vi "PrepareGameData.vi"(8 "error in":errorcluster, 11 "GameDataIn":T1) -> (0 "error out":errorcluster, 3 "GameDataOut":T1)   [LabVIEW 2024]
uses:
  Controls/ArmySelector.ctl
  Controls/GameInfo.ctl
  Controls/E_Phases.ctl
  <vilib>/Utility/file.llb/Read Delimited Spreadsheet (string).vi
panel:
  in  "Opponent Army":T3
  in  "Player Army":T3
  out "String":string
  in  "Done":bool
  in  "LocationOfData":path
  in  "OpponentName":string
  in  "PlayerName":string
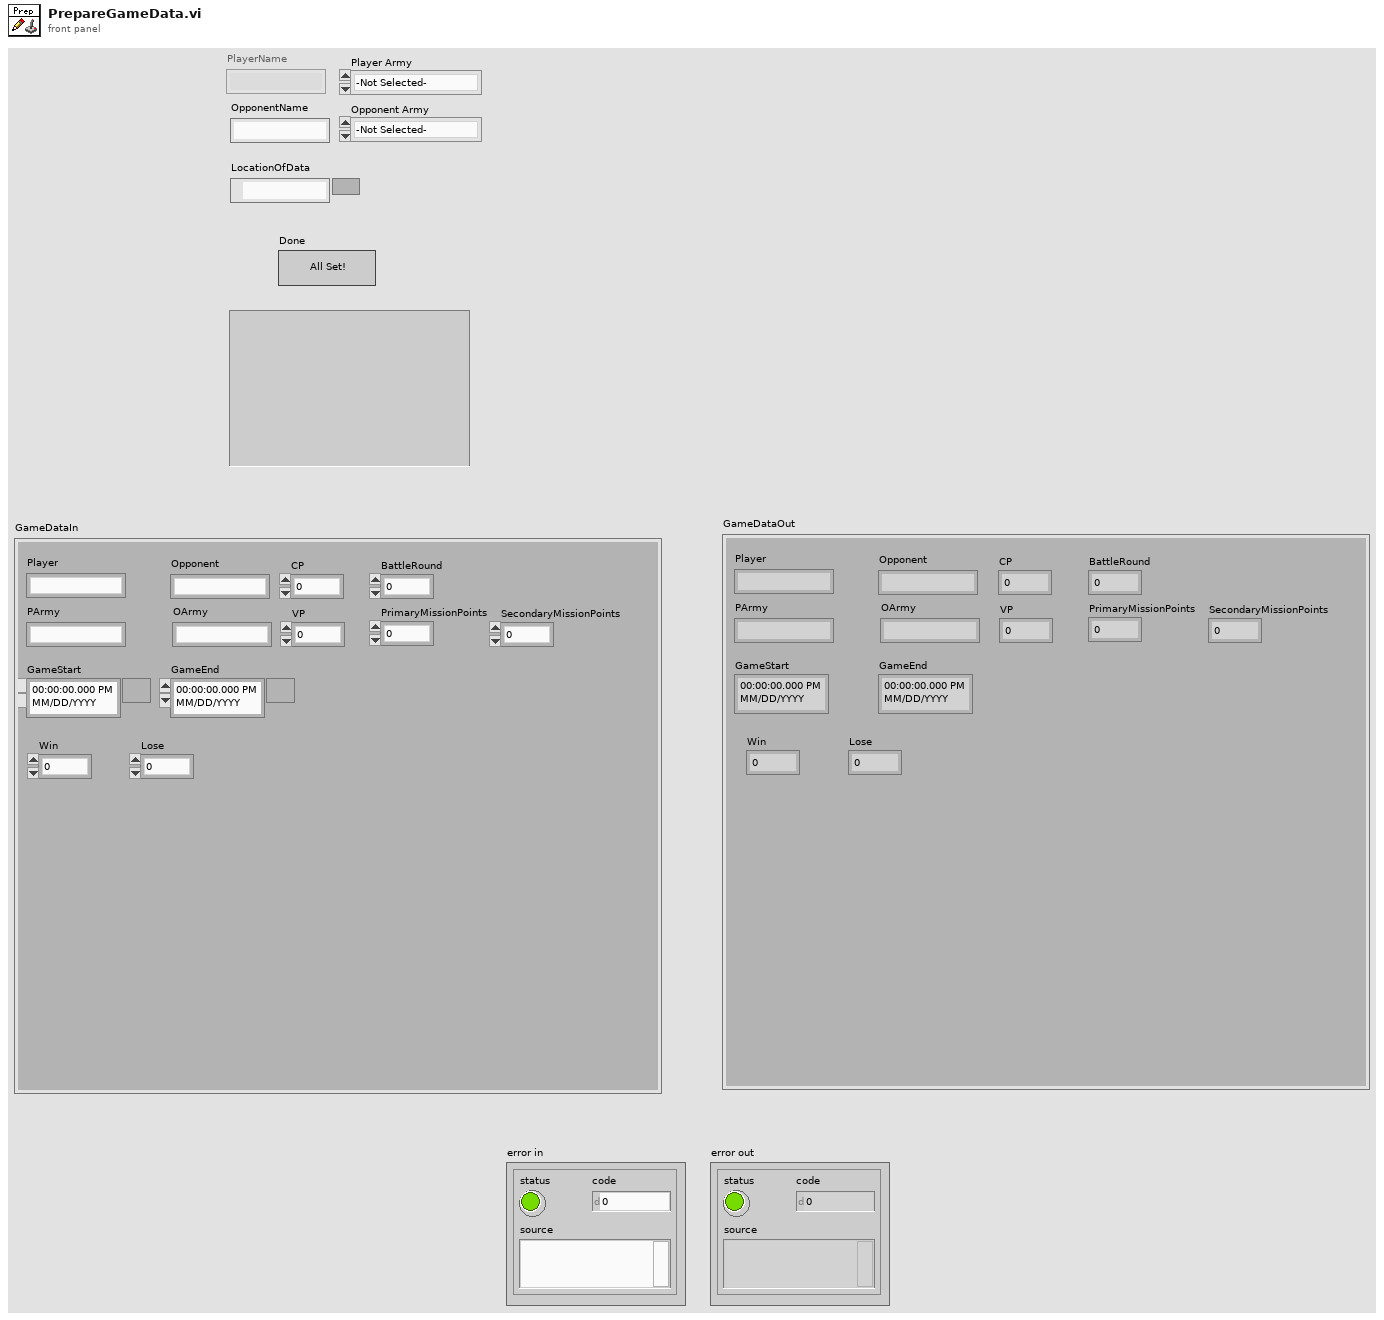
[diagram p1: front panel]
types:
  T1 = typedef "GameInfo.ctl" = cluster{"Player":string, "Opponent":string, "PArmy":string, "OArmy":string, "CP":dbl, "VP":dbl, "GameStart":timestamp, "GameEnd":timestamp, "BattleRound":dbl, "PrimaryMissionPoints":dbl, "SecondaryMissionPoints":dbl, "BattlePhase":T2, "Win":dbl, "Lose":dbl}
  T2 = typedef "E_Phases.ctl" = enum16{"Null/Error", "Command Phase", "Movement Phase", "Shooting Phase", "Charge Phase", "Fight Phase", "Secondary Scoring", "Enemy Command Phase", "Enemy Movement Phase", "Enemy Shooting Phase", "Enemy Charge Phase", "Enemy Fight Phase", "Enemy Secondary Scoring"}
  T3 = typedef "ArmySelector.ctl" = enum16{"-Not Selected-", "Adepta Sororitas", "Dark Angels", "T'au Empire", "Necrons"}
  T4 = enum8{"Enabled", "Disabled", "Disabled and Grayed Out"}
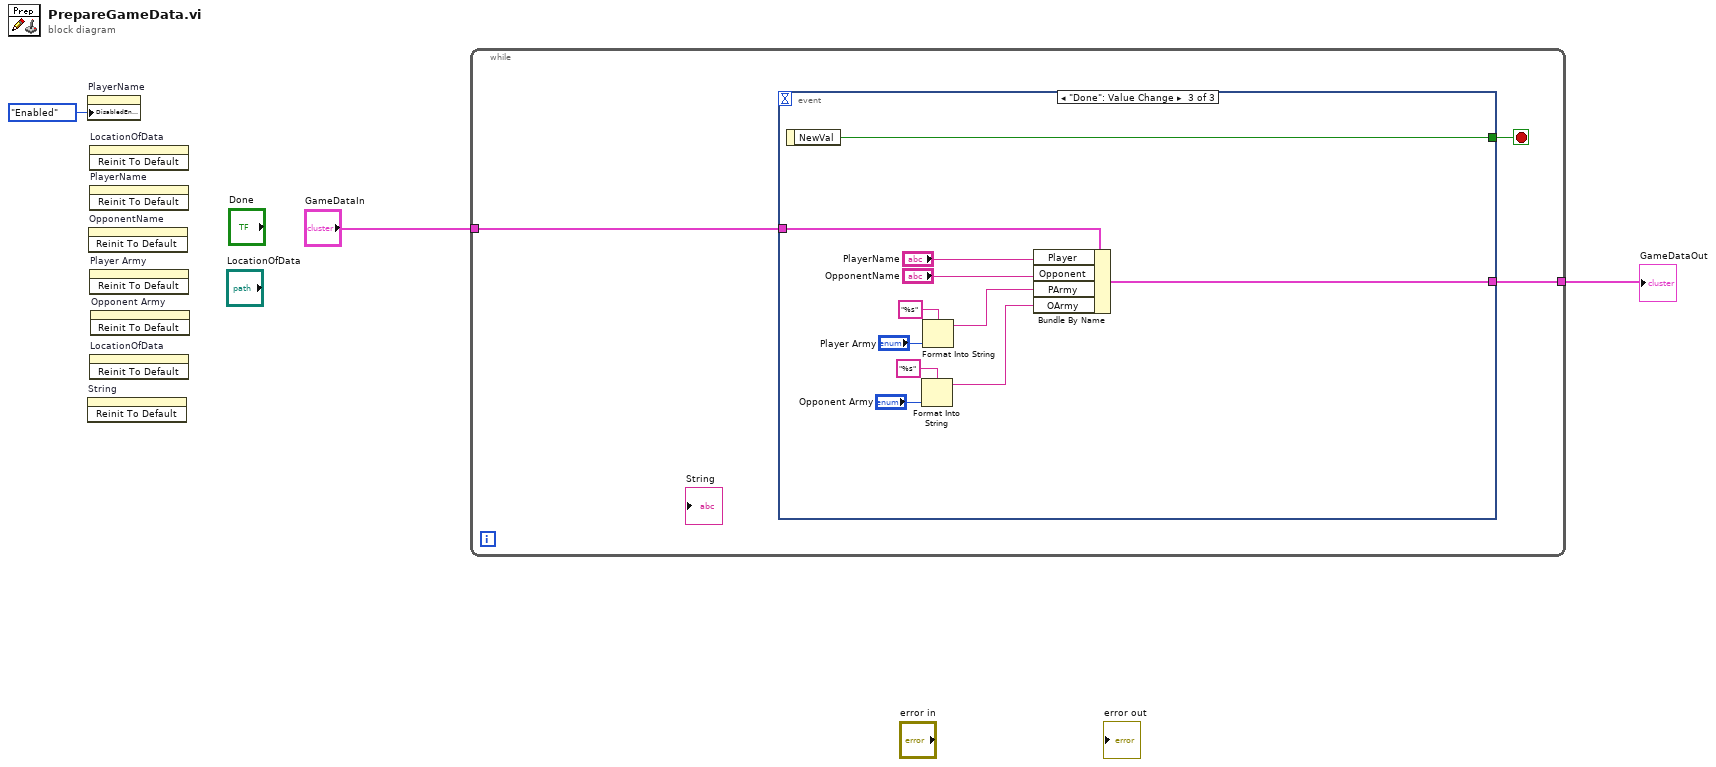
[diagram p0: block diagram]
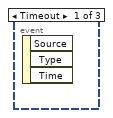
[diagram p2: hidden frame]
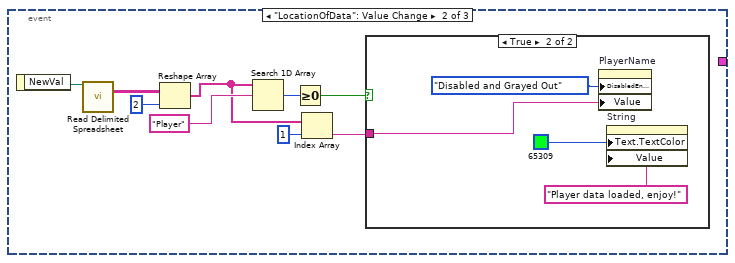
[diagram p3: hidden frame]
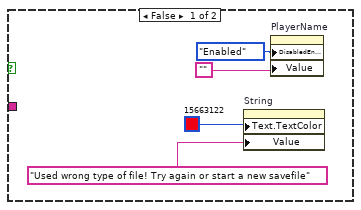
[diagram p4: hidden frame]
diagram:
  n1 = property on="PlayerName" class="Str"("DisabledEnum"=T4."Enabled" ("Disabled")) -> ()  [unwired: 2 in, 2 out]
  n2 = invoke on="String" class="Str" method="Reinit To Default"() -> ()  [unwired: 3 in, 3 out]
  n3 = invoke on="OpponentName" class="Str" method="Reinit To Default"() -> ()  [unwired: 3 in, 3 out]
  n4 = invoke on="LocationOfData" class="Path" method="Reinit To Default"() -> ()  [unwired: 3 in, 3 out]
  n5 = invoke on="PlayerName" class="Str" method="Reinit To Default"() -> ()  [unwired: 3 in, 3 out]
  n6 = invoke on="Player Army" class="Enum (strict)" method="Reinit To Default"() -> ()  [unwired: 3 in, 3 out]
  n7 = invoke on="LocationOfData" class="Path" method="Reinit To Default"() -> ()  [unwired: 3 in, 3 out]
  n8 = invoke on="Opponent Army" class="Enum (strict)" method="Reinit To Default"() -> ()  [unwired: 3 in, 3 out]
  n9 = while {
    tunnel: "GameDataIn" -> [w5]
    tunnel: [w4] -> w1
    stop <- w6 stop-if-true
    n10 = event shown="[2] \"Done\": Value Change" {
      selector: _ -> [_ _ _]
      dyn-events: _ -> [_ _ _]
      timeout: _ -> [_ _ _]
      tunnel: [_ _ w34] -> w6
      tunnel: w5 -> [_ _ w33]
      tunnel: [_ _ w24] -> w4
      event Timeout {
        n11 = event-data() -> ()  [unwired: 1 in, 3 out]
      }
      event "LocationOfData": Value Change {
        n12 = event-data() -> ("NewVal"=w7:path)  [unwired: 1 in]
        n13 = call-poly <vilib>:"Read Delimited Spreadsheet.vi"("file path (dialog if empty)"=w7) -> ("all rows"=w15:string[][])  [unwired: 9 in, 5 out]
        n14 = Reshape Array(w15, 2 ("dimension size")) -> (w11:string[])
        n15 = Search 1D Array(1D array=w11, element="Player") -> (index of element=w10:i32)  [unwired: 1 in]
        n16 = Greater Or Equal To 0?(x=w10) -> (x >= 0?=w12:bool)
        n17 = Index Array(array=w11, index=1) -> (element=w9:string)
        n18 = case shown="True" w12 {
          tunnel: w9 -> [_ w22]
          frame False {
            n19 = property on="String" class="Str"("Text.TextColor"=u32 15663122, "Value"="Used wrong type of file! Try again or start a new savefile" ("String")) -> ()  [unwired: 2 in, 2 out]
            n20 = property on="PlayerName" class="Str"("DisabledEnum"=T4."Enabled" ("Disabled"), "Value"="") -> ()  [unwired: 2 in, 2 out]
          }
          frame True {
            n21 = property on="PlayerName" class="Str"("DisabledEnum"=T4."Disabled and Grayed Out" ("Disabled"), "Value"=w22) -> ()  [unwired: 2 in, 2 out]
            n22 = property on="String" class="Str"("Text.TextColor"=u32 65309, "Value"="Player data loaded, enjoy!" ("String")) -> ()  [unwired: 2 in, 2 out]
          }
        }
      }
      event "Done": Value Change {
        n23 = event-data() -> ("NewVal"=w34:bool)  [unwired: 1 in]
        n24 = Format Into String(format string="%s", "Opponent Army") -> (resulting string=w25:string)  [unwired: 2 in, 1 out]
        n25 = Format Into String(format string="%s", "Player Army") -> (resulting string=w26:string)  [unwired: 2 in, 1 out]
        n26 = Bundle By Name(cluster=w33, "Player"="PlayerName", "Opponent"="OpponentName", "PArmy"=w26, "OArmy"=w25) -> (w24:T1)
      }
    }
  }
  "GameDataOut" <- w1
